vi "POSiReadout.vi"(1 "Resource Name 0":refnum<visa-resource-name>="COM9") -> (0 "Position number":i32)   [LabVIEW 2012]
uses:
  <vilib>/Instr/_visa.llb/VISA Configure Serial Port (Instr).vi
panel:
  out "POSItion":string
  out "Error Out":errorcluster={"status"=TRUE, "code"=-1073807343, "source"="VISA Write in Serial Communication for TL3T of VISA.vi"}
  out "concatenated string":string="@0X2000,\r\n"
  in  "baud rate (9600)":u32=9600
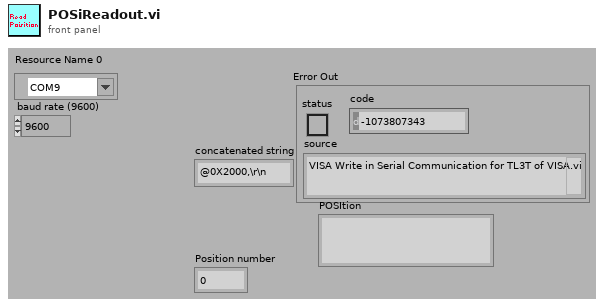
[diagram p1: front panel]
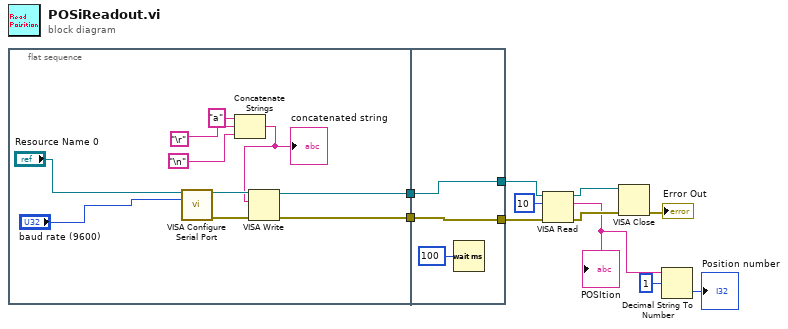
[diagram p0: block diagram]
diagram:
  n1 = flat-sequence {
    tunnel: [w14] -> w9
    tunnel: [w13] -> w7
    tunnel: [w24] -> w10
    tunnel: w9 -> [w24]
    tunnel: [w22] -> w8
    tunnel: w7 -> [w22]
    frame #0 {
      n2 = call-poly "VISA Configure Serial Port"("VISA resource name"="Resource Name 0", "baud rate (9600)"="baud rate (9600)") -> ("VISA resource name out"=w19:refnum<visa-resource-name>, "error out"=w15:errorcluster)  [unwired: 12 in]
      n3 = Concatenate Strings("a" ("string"), "\r", "\n") -> (w16:string)
      "concatenated string" <- w16
      n4 = VISA Write(VISA resource name=w19, write buffer=w16, error in (no error)=w15) -> (VISA resource name out=w14:refnum<visa-resource-name>, error out=w13:errorcluster)  [unwired: 1 out]
    }
    frame #1 {
      n5 = Wait (ms)(milliseconds to wait=u32 100) -> ()  [unwired: 1 out]
    }
  }
  n6 = VISA Read(VISA resource name=w10, byte count=u32 10, error in (no error)=w8) -> (VISA resource name out=w4:refnum<visa-resource-name>, read buffer=w3:string, error out=w5:errorcluster)  [unwired: 1 out]
  "POSItion" <- w3
  n7 = VISA Close(VISA resource name=w4, error in (no error)=w5) -> (error out=→"Error Out":errorcluster)
  n8 = Decimal String To Number(string=w3, offset=1) -> (number=→"Position number":i32)  [unwired: 1 in, 1 out]
